vi "Leak check durchfuehren.vi"(8 "TablePictures Refnum In":refnum<vi>[](array[refnum]), 9 "Temperatur":sgl, 10 "Druck FT-IR":sgl, 11 "Aktion":T1) -> (0 "Verstrichene Zeit":sgl, 1 "Druckanstieg":sgl, 2 "Status":string, 3 "Aktion":T1, 4 "Fehler":bool, 5 "Fertig":bool)   [LabVIEW 2020, in "EPA 1065.lvlib" / "Dichtheitstest 1065-345.lvlib"]
uses:
  Dichtheitstest 1065-345.lvlib
  Aktion Leak check durchfuehren.ctl
  Aktion Leak Daten.ctl
  Aktion Protokolldaten_Leak check.ctl
  Sprachverwaltung/FGV Aktion Tabelle zerlegen.ctl
  Funktionstasten/Freigabe Aktionen.ctl
  PNS/Aktionen FGV Grenzwerte.ctl
  Funktionstasten/Zustaende.ctl
  Funktionstasten/Funktionstasten-Aktion.ctl
  Stoerungen/Stoerungen Messgeraet/Aktionen Kommunikation Stoerung.ctl
  Aktion FGV Automatic start.ctl
  Leak Daten.ctl
  Seiten/FT-IR/FT-IR.lvlib
  Stoerungen/Stoerungen.lvlib
  PNS/PNS.lvlib
  Funktionstasten/Funktionstasten.lvlib
  Sprachverwaltung/Sprachverwaltung.lvlib
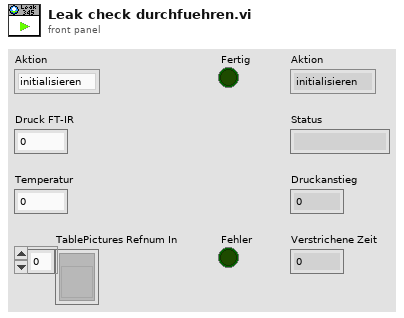
[diagram p1: front panel]
types:
  T1 = typedef "EPA 1065.lvlib/Dichtheitstest 1065-345.lvlib/Aktion Leak check durchfuehren.ctl" = enum16{"initialisieren", "Unterdruck erzeugen", "Ventile schließen", "Warten", "Auswertung", "fertig", "PDF erstellen", "abbrechen"}
  T2 = typedef "EPA 1065.lvlib/Dichtheitstest 1065-345.lvlib/Aktion Leak Daten.ctl" = enum16{"lesen", "laden", "speichern", "Volumen", "berechnen", "Leak check aktiv", "Leak Zustand", "Pfad", "Pfad speichern"}
  T3 = typedef "PNS.lvlib/Aktionen FGV Grenzwerte.ctl" = enum16{"lesen", "Grenzw. schreiben", "Anweisungscode", "IP-Adresse", "laden", "speichern", "Anweisungscode vorgeben"}
  T4 = typedef "Funktionstasten.lvlib/Freigabe Aktionen.ctl" = enum16{"prüfen", "Freigabe?", "lesen"}
  T5 = typedef "Sprachverwaltung.lvlib/FGV Aktion Tabelle zerlegen.ctl" = enum16{"laden", "vereinzeln", "speichern"}
  T6 = typedef "EPA 1065.lvlib/Dichtheitstest 1065-345.lvlib/Aktion Protokolldaten_Leak check.ctl" = enum16{"lesen", "Zeitstempel", "Bearbeiter", "Daten", "Auswertung", "löschen"}
  T7 = typedef "Funktionstasten.lvlib/Funktionstasten-Aktion.ctl" = enum16{"Initialisieren", "Zustand setzen", "Taste gedrückt", "Fehler speichern", "Lesen", "Manuell", "Remote", "Bitparallel", "Samplepoint", "Zeit Prüfen", "reset Umschalten"}
  T8 = typedef "Funktionstasten.lvlib/Zustaende.ctl" = enum16{"Standby", "Pause", "Eco", "Messen", "Kalibrieren", "Spülen Filter", "Spülen Leitung", "Umgebungsluft", "0-Gas", "Cal-Gas", "CG zu PNS", "-------------", "Init 1", "Init 2", "Init 3", "Init 4", "Messen vorbereiten", "Messen durchführen", "Exit"}
  T9 = typedef "EPA 1065.lvlib/Dichtheitstest 1065-345.lvlib/Leak Daten.ctl" = cluster{"Gesamtes Volumen":sgl, "p 1":sgl, "p 2":sgl, "T 1":sgl, "T 2":sgl, "t 1":timestamp, "t 2":timestamp, "Ergebnis mol/s":sgl, "Grenze mol/s":sgl, "Leak in %":sgl, "Ergebnis mbar":sgl, "Grenze mbar":sgl}
  T10 = typedef "EPA 1065.lvlib/Dichtheitstest 1065-345.lvlib/Aktion FGV Automatic start.ctl" = enum16{"lesen", "Test starten aktiv", "Test starten inaktiv", "Seite merken", "Seite zurücksetzen", "AK Start inaktiv"}
  T11 = typedef "Stoerungen.lvlib/Aktionen Kommunikation Stoerung.ctl" = enum16{"lesen", "init", "FT-IR Komm", "FT-IR Betriebsart", "FT-IR Hintergrund", "cRIO Komm", "PNS Komm", "Dichtheitstest", "Life Bit", "FTIR Komm AK", "PMA Komm", "FID Komm", "PMA Cal", "FID Ch4 Cal", "FID THC Cal", "Cal Timeout", "VFS 1 Komm", "VFS 2 Komm", "VFS 3 Komm", "VFS 4 Komm", "TRE 08 Komm", "CG-Test vorzeitig", "CG-Test Span 1", "CG-Test Span 2", "CG-Test Span 3", "CG-Test Messgas", "CG-Test löschen", "Test", "Amium AK", "AK Recept konfig", "AK Name konfig", "AK EKFG konfig"}
  T12 = typedef "EPA 1065.lvlib/Dichtheitstest 1065-345.lvlib/Gesamtvolumen.ctl" = cluster{"FAS":sgl, "d von HL zu VFS":sgl, "l von HL zu VFS":sgl, "VFS":sgl, "d von HL zu SP":sgl, "l von HL zu SP":sgl, "Heizleitung zum VFS":bool, "VFS a":bool, "Heizleitung zur Entnahmestelle":bool, "Gesamtes Volumen":sgl, "LeakValve":u16, "Einheit":enum16{"mol/s", "mbar"}}
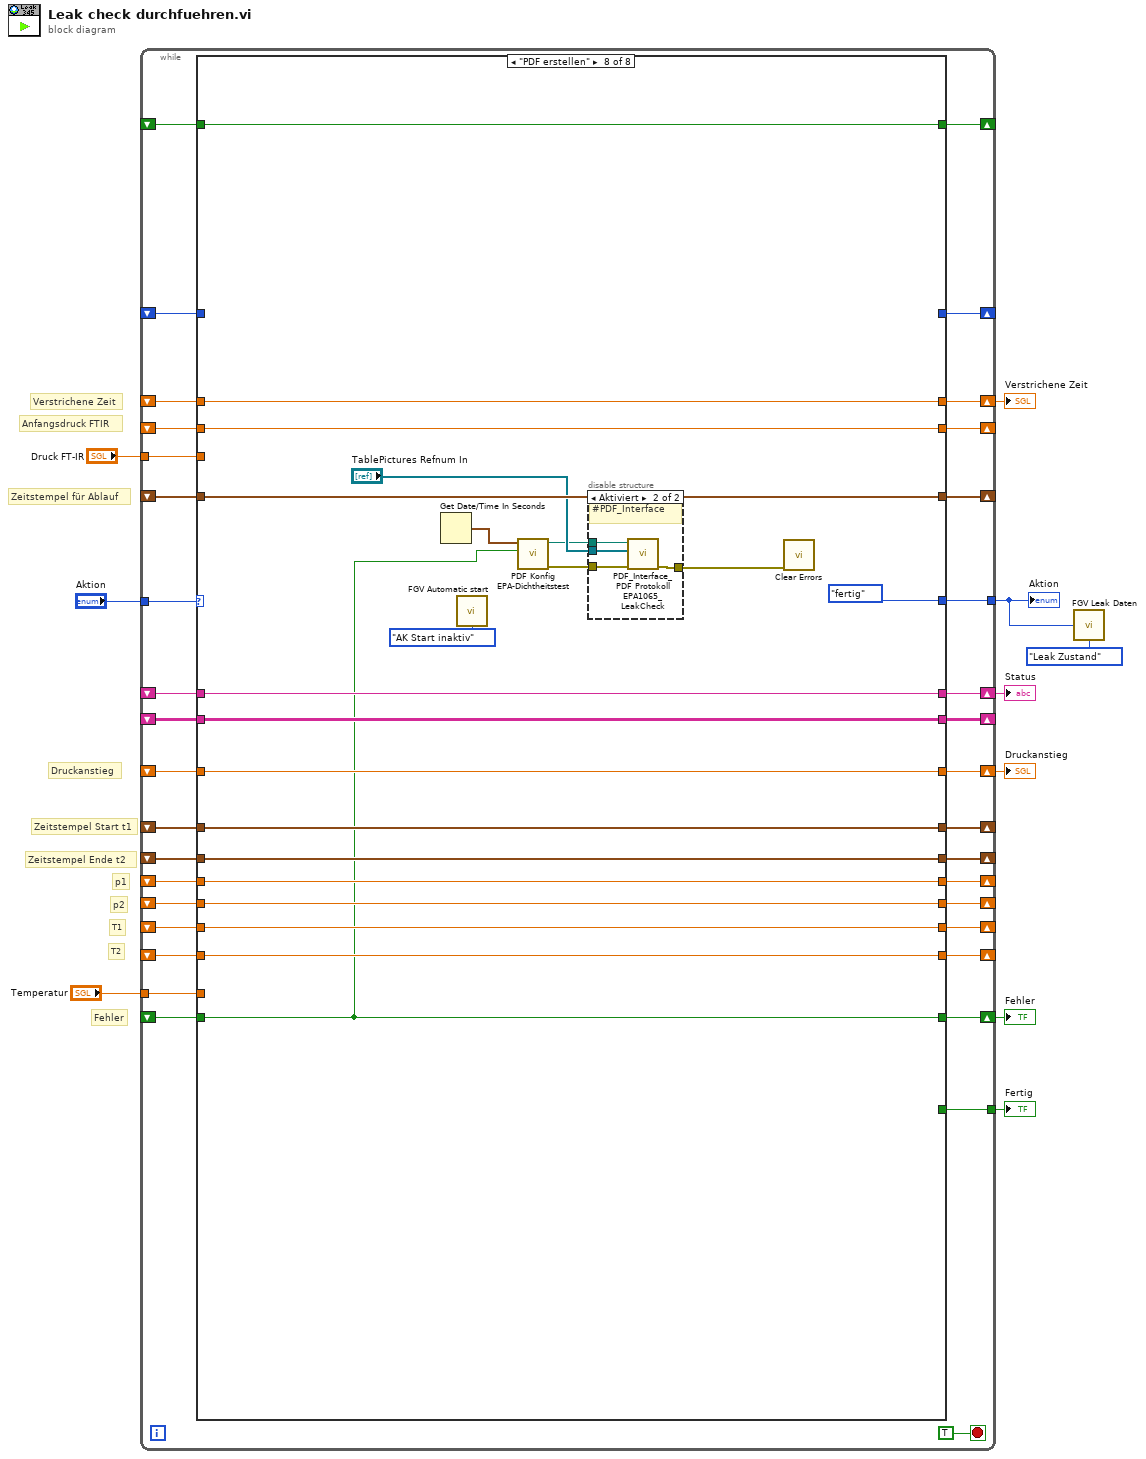
[diagram p0: block diagram]
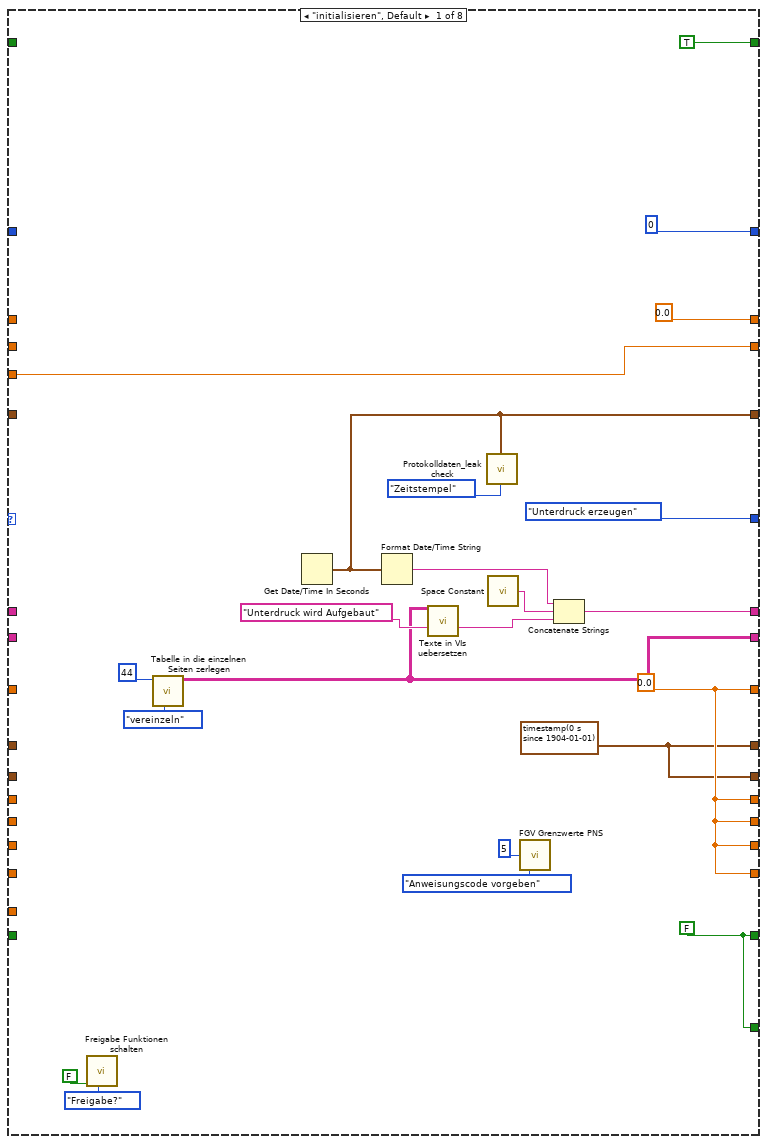
[diagram p2: hidden frame]
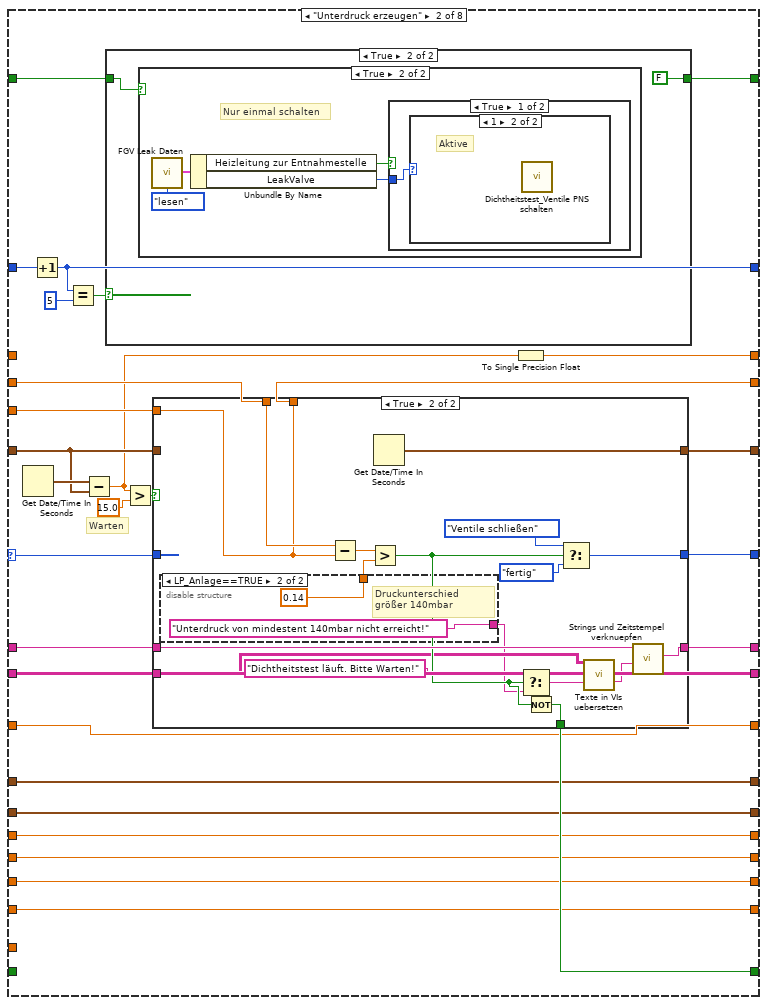
[diagram p3: hidden frame]
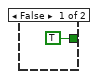
[diagram p4: hidden frame]
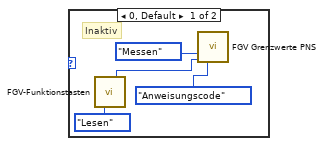
[diagram p6: hidden frame]
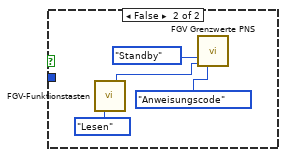
[diagram p7: hidden frame]
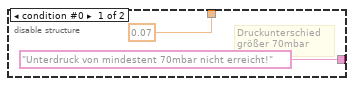
[diagram p9: hidden frame]
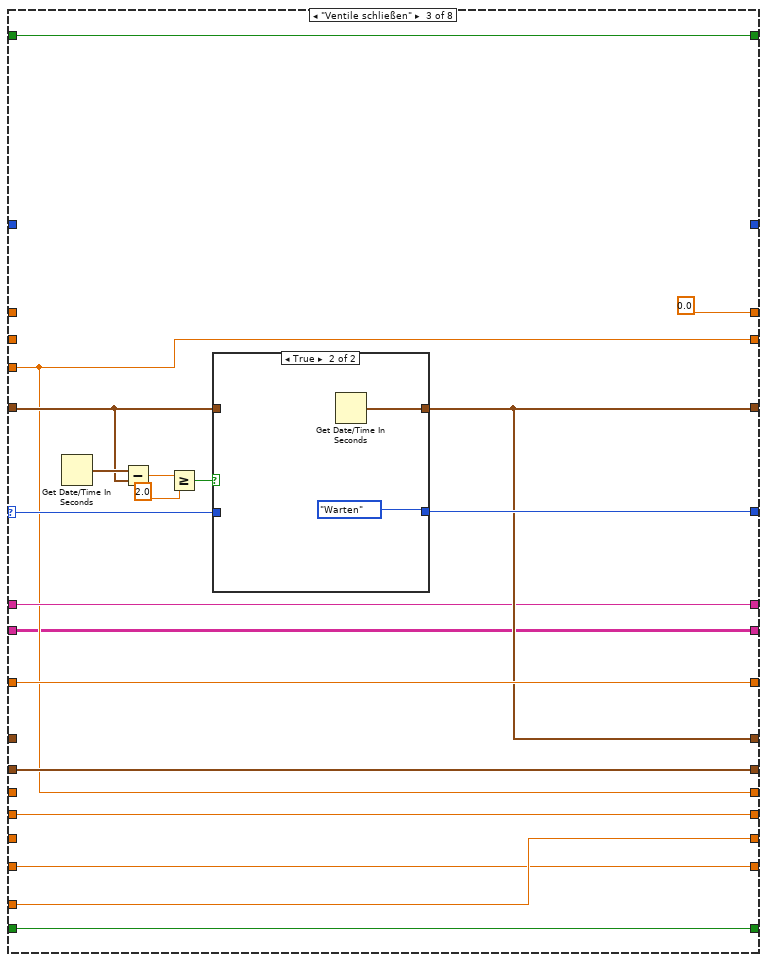
[diagram p10: hidden frame]
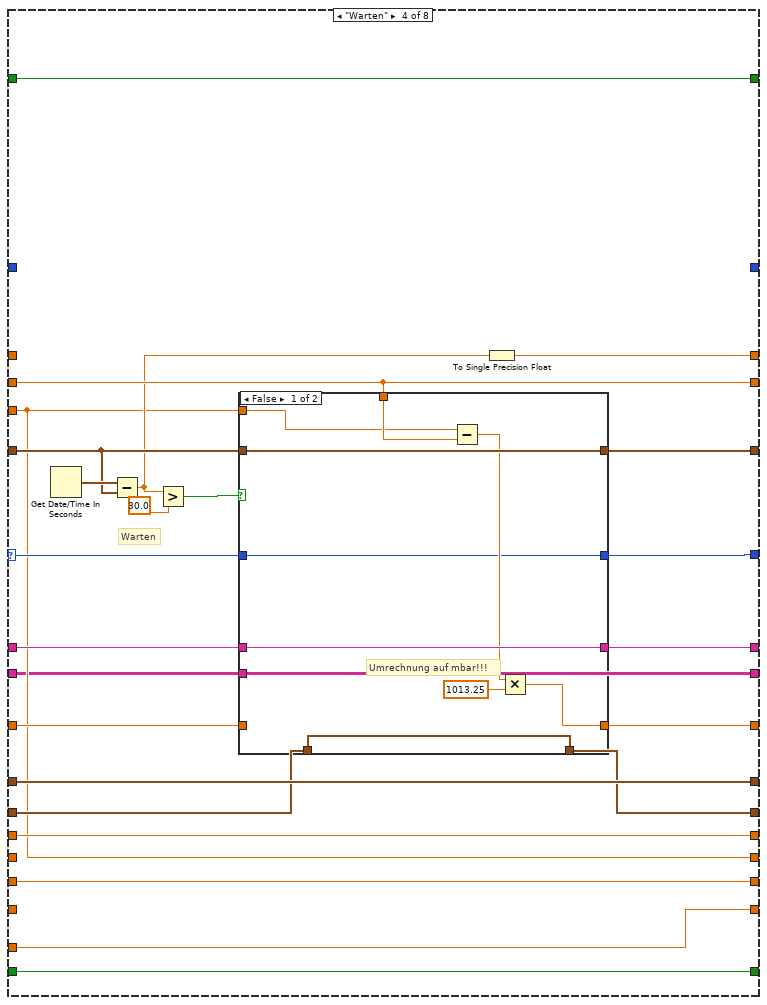
[diagram p12: hidden frame]
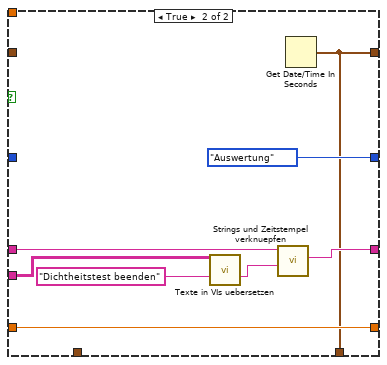
[diagram p13: hidden frame]
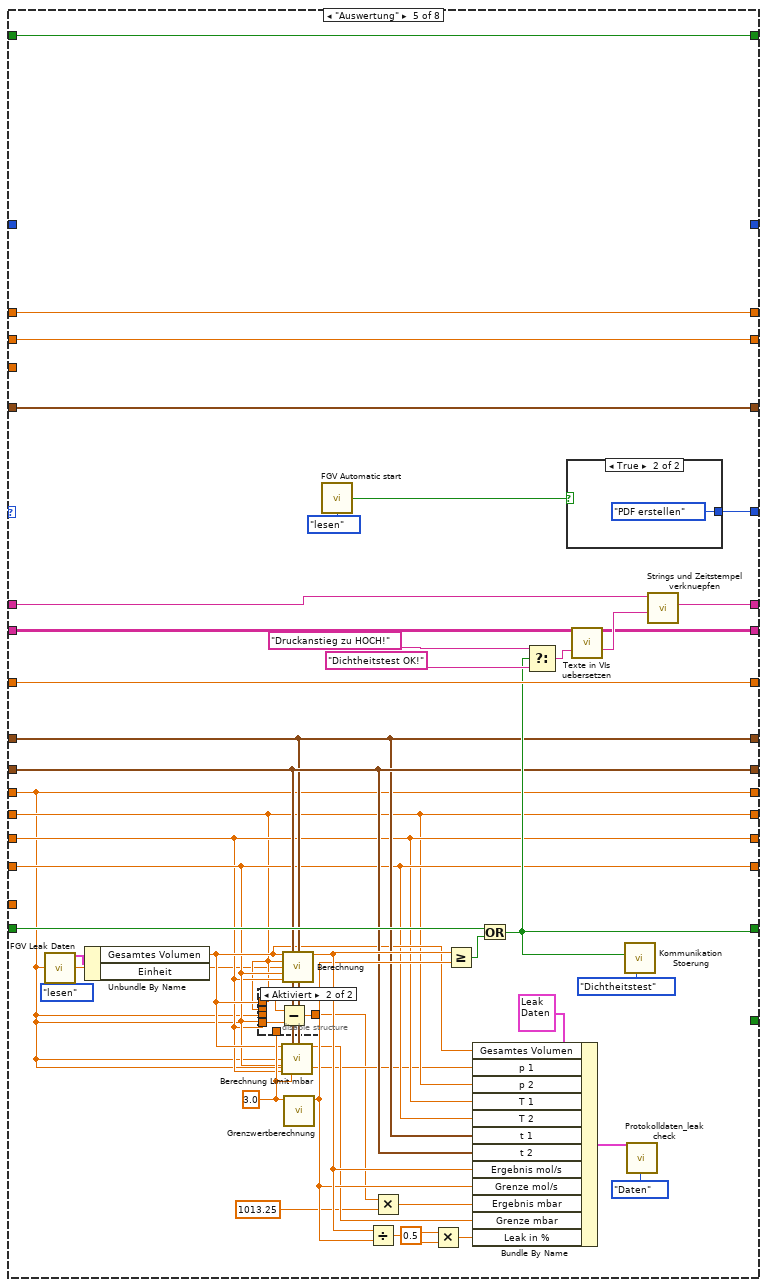
[diagram p14: hidden frame]
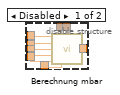
[diagram p15: hidden frame]
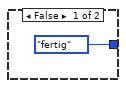
[diagram p16: hidden frame]
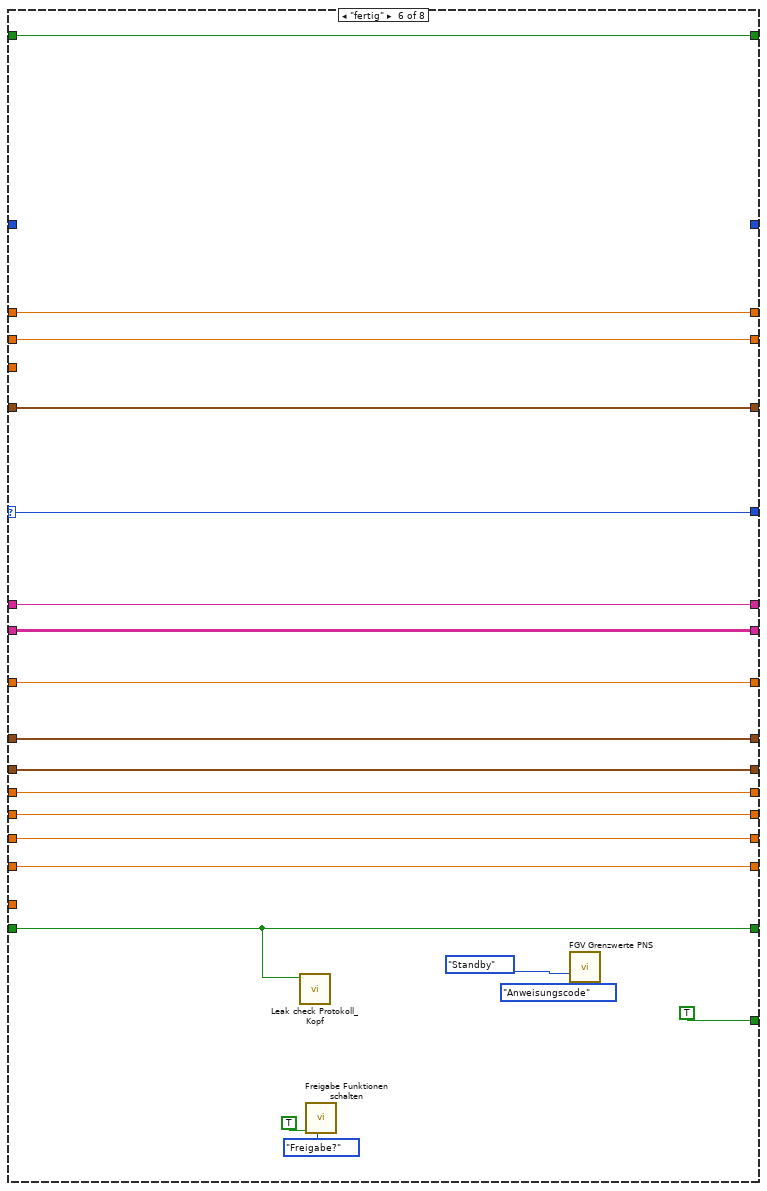
[diagram p17: hidden frame]
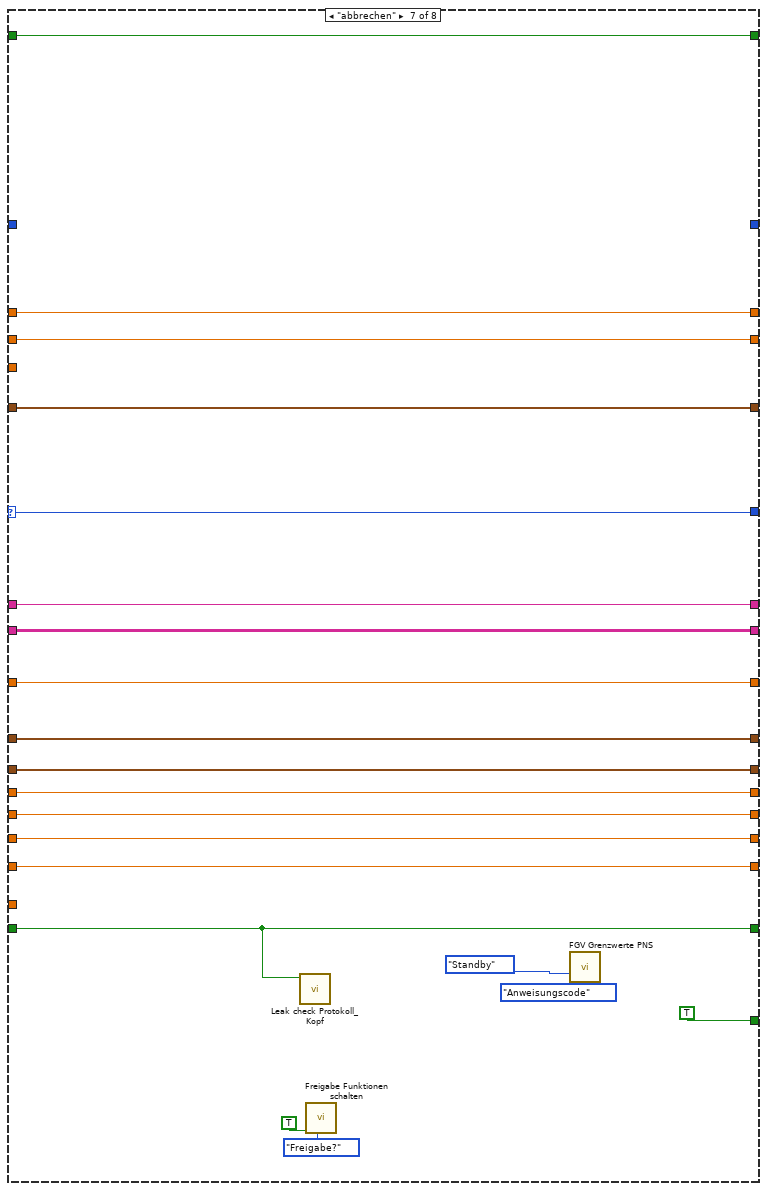
[diagram p18: hidden frame]
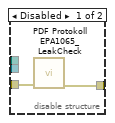
[diagram p19: hidden frame]
diagram:
  # "T2"
  # "T1"
  # "p2"
  # "p1"
  # "Druckanstieg"
  # "Zeitstempel Ende t2"
  # "Zeitstempel Start t1"
  # "Fehler"
  # "Zeitstempel für Ablauf"
  # "Verstrichene Zeit"
  # "Anfangsdruck FTIR"
  n1 = while {
    shift-right: [w44] -> _
    shift-left: _ -> [w42]
    shift-right: [w41] -> w8
    shift-left: _ -> [w40]
    tunnel: "Aktion" -> [w45]
    tunnel: [w43] -> w1
    tunnel: "Druck FT-IR" -> [w39]
    shift-right: [w38] -> _
    shift-left: _ -> [w37]
    shift-right: [w36] -> w6
    shift-left: _ -> [w35]
    shift-right: [w34] -> w4
    shift-left: _ -> [w33]
    shift-right: [w32] -> w5
    shift-left: _ -> [w31]
    shift-right: [w30] -> _
    shift-left: _ -> [w29]
    shift-right: [w27] -> _
    shift-left: _ -> [w28]
    shift-right: [w26] -> _
    shift-left: _ -> [w25]
    shift-right: [w24] -> _
    shift-left: _ -> [w23]
    tunnel: "Temperatur" -> [w22]
    shift-right: [w21] -> _
    shift-left: _ -> [w20]
    shift-right: [w19] -> _
    shift-left: _ -> [w18]
    tunnel: [w17] -> w3
    shift-right: [w16] -> _
    shift-left: _ -> [w15]
    shift-right: [w14] -> _
    shift-left: _ -> [w13]
    shift-right: [w12] -> _
    shift-left: _ -> [w11]
    stop <- TRUE stop-if-true
    n2 = case shown="\"PDF erstellen\"" w45 {
      selector: w45 -> [_ w90 w152 w178 _ w274 w294 _]
      tunnel: [w58 w97 w150 w184 w241 w275 w295 w316] -> w44
      tunnel: [Aktion_Leak_check_durchfuehren."Unterdruck erzeugen" ("Aktion") w89 w151 w177 w238 w274 w294 Aktion_Leak_check_durchfuehren."fertig" ("Aktion")] -> w43
      tunnel: w42 -> [_ w93 w153 w182 w241 w275 w295 w316]
      tunnel: [w65 w92 w147 w175 w232 w273 w293 w314] -> w41
      tunnel: w40 -> [_ w91 w147 w176 w233 w273 w293 w314]
      tunnel: w39 -> [w64 w88 w145 w167 _ _ _ _]
      tunnel: [w64 w86 w145 w180 w240 w276 w296 w317] -> w38
      tunnel: w37 -> [_ w87 _ w180 w240 w276 w296 w317]
      tunnel: [sgl 0.0 w77 sgl 0.0 w164 w239 w277 w297 w318] -> w36
      tunnel: w35 -> [_ _ _ _ w239 w277 w297 w318]
      tunnel: [w60 w85 w141 w169 w229 w262 w282 w302] -> w34
      tunnel: w33 -> [_ _ w141 w169 w234 w262 w282 w302]
      tunnel: [w62 w82 w157 w174 w242 w272 w292 w312] -> w32
      tunnel: w31 -> [_ w82 w157 w173 w242 w272 w292 w312]
      tunnel: [w61 w84 w150 w172 w212 w271 w291 w311] -> w30
      tunnel: w29 -> [_ w84 _ w172 w212 w271 w291 w311]
      tunnel: w28 -> [_ w83 w149 w170 w213 w270 w290 w310]
      tunnel: [w61 w83 w149 w171 w213 w270 w290 w310] -> w27
      tunnel: [w62 w81 w145 w168 w206 w269 w289 w309] -> w26
      tunnel: w25 -> [_ w81 _ w168 w206 w269 w289 w309]
      tunnel: [w62 w80 w143 w167 w207 w268 w288 w308] -> w24
      tunnel: w23 -> [_ w80 w143 _ w207 w268 w288 w308]
      tunnel: w22 -> [_ _ w144 w166 _ _ _ _]
      tunnel: [w62 w78 w142 w166 w210 w266 w286 w306] -> w21
      tunnel: w20 -> [_ w78 w142 _ w210 w266 w286 w306]
      tunnel: [w62 w79 w144 w165 w209 w267 w287 w307] -> w19
      tunnel: w18 -> [_ w79 _ w165 w209 w267 w287 w307]
      tunnel: [w60 _ _ _ _ TRUE TRUE _] -> w17
      tunnel: [w54 w76 w140 w163 w225 w261 w281 w313] -> w16
      tunnel: w15 -> [_ w76 w140 w163 w225 w261 w281 w313]
      tunnel: [0 w73 _ _ _ _ _ _] -> w14
      tunnel: w13 -> [_ w74 _ _ _ _ _ _]
      tunnel: [TRUE w70 w139 w162 w220 w258 w278 w300] -> w12
      tunnel: w11 -> [_ w69 w139 w162 w220 w258 w278 w300]
      frame "initialisieren", Default {
        w60 = FALSE
        w61 = timestamp(0 s since 1904-01-01) ("seconds since 1Jan1904")
        w62 = sgl 0.0
        n3 = call "Freigabe Funktionen schalten.vi"("Aktionen"=Freigabe_Aktionen."Freigabe?", "Freigabe?"=FALSE) -> ()  [unwired: 7 in, 3 out]
        n4 = call "Tabelle in die einzelnen Seiten zerlegen.vi"("Aktion"=FGV_Aktion_Tabelle_zerlegen."vereinzeln", "Index (Seite)"=44) -> ("Sprachliste"=w54:string[][])  [unwired: 7 in, 2 out]
        n5 = Get Date/Time In Seconds() -> (seconds since 1Jan1904=w58:timestamp)
        n6 = Format Date/Time String(seconds (now)=w58) -> (date/time string=w68:string)  [unwired: 2 in]
        n7 = call "Texte in VIs uebersetzen.vi"("Sprachliste"=w54, "String zum Übersetzen"="Unterdruck wird Aufgebaut" ("String")) -> ("String zum Übersetzen"=w55:string)  [unwired: 9 in, 4 out]
        n8 = call "Protokolldaten_leak check.vi"("Start"=w58, "Aktion"=Aktion_Protokolldaten_Leak_check."Zeitstempel") -> ()  [unwired: 22 in, 4 out]
        n9 = call <vilib>:"Space Constant.vi"() -> ("String"=w67:string)
        n10 = call "FGV Grenzwerte PNS.vi"("Anweisungscode"=u16 5, "Aktionen FGV Grenzwerte"=Aktionen_FGV_Grenzwerte."Anweisungscode vorgeben") -> ()  [unwired: 11 in, 3 out]
        n11 = Concatenate Strings(w68, w67, w55) -> (w65:string)
      }
      frame "Unterdruck erzeugen" {
        # "Warten"
        n12 = Get Date/Time In Seconds() -> (seconds since 1Jan1904=w95:timestamp)
        n13 = Increment(x=w74) -> (x+1=w73:i32)
        n14 = Equal?(x=w73, y=5) -> (x = y?=w71:bool)
        n15 = Subtract(x=w95, y=w93) -> (x-y=w75:dbl)
        n16 = case shown="True" w71 {
          tunnel: [TRUE FALSE] -> w70
          tunnel: w69 -> [_ w99]
          frame False {
          }
          frame True {
            n17 = case shown="True" w99 {
              frame False {
              }
              frame True {
                # "Nur einmal schalten"
                n18 = call "FGV Leak Daten.vi"("Aktion"=Aktion_Leak_Daten."lesen") -> ("Gesamtvolumen"=w103:T12)  [unwired: 10 in, 4 out]
                n19 = Unbundle By Name(w103) -> ("Heizleitung zur Entnahmestelle"=w102:bool, "LeakValve"=w101:u16)
                n20 = case shown="True" w102 {
                  tunnel: w101 -> [w105 _]
                  frame True {
                    n21 = case shown="1" w105 {
                      frame 0, Default {
                        # "Inaktiv"
                        n22 = call "FGV-Funktionstasten.vi"("Aktion"=Funktionstasten-Aktion."Lesen") -> ("Samplepoint"=w106:u16)  [unwired: 7 in, 7 out]
                        n23 = call "FGV Grenzwerte PNS.vi"("Zustand"=Zustaende."Messen", "Samplepoint"=w106, "Aktionen FGV Grenzwerte"=Aktionen_FGV_Grenzwerte."Anweisungscode") -> ()  [unwired: 10 in, 3 out]
                      }
                      frame 1 {
                        # "Aktive"
                        n24 = call "Dichtheitstest_Ventile PNS schalten.vi"() -> ()  [unwired: 11 in, 1 out]
                      }
                    }
                  }
                  frame False {
                    n25 = call "FGV-Funktionstasten.vi"("Aktion"=Funktionstasten-Aktion."Lesen") -> ("Samplepoint"=w110:u16)  [unwired: 7 in, 7 out]
                    n26 = call "FGV Grenzwerte PNS.vi"("Zustand"=Zustaende."Standby", "Samplepoint"=w110, "Aktionen FGV Grenzwerte"=Aktionen_FGV_Grenzwerte."Anweisungscode") -> ()  [unwired: 10 in, 3 out]
                  }
                }
              }
            }
          }
        }
        n27 = Greater?(x=w75, y=15.0) -> (0:w94:bool)
        n28 = case shown="True" w94 {
          tunnel: w93 -> [w117 _]
          tunnel: [w117 w122] -> w97
          tunnel: w87 -> [w116 w134]
          tunnel: [w116 w125] -> w86
          tunnel: [w115 w131] -> w89
          tunnel: w91 -> [w114 w130]
          tunnel: [w114 w129] -> w92
          tunnel: w90 -> [w115 _]
          tunnel: [_ w126] -> w85
          tunnel: w88 -> [_ w125]
          tunnel: w76 -> [_ w119]
          frame False {
          }
          frame True {
            n29 = disable-structure shown="LP_Anlage==TRUE" {
              disable-tunnel: [0.07 ("y") 0.14 ("y")] -> w132
              disable-tunnel: ["Unterdruck von mindestent 70mbar nicht erreicht!" ("String") "Unterdruck von mindestent 140mbar nicht erreicht!" ("String")] -> w118
              frame condition #0 {
                # "Druckunterschied \ngrößer 70mbar"
              }
              frame condition #1 (active) {
                # "Druckunterschied \ngrößer 140mbar"
              }
            }
            n30 = Subtract(x=w134, y=w125) -> (x-y=w133:sgl)
            n31 = Greater?(x=w133, y=w132) -> (0:w127:bool)
            n32 = Get Date/Time In Seconds() -> (seconds since 1Jan1904=w122:timestamp)
            n33 = Select(t="Dichtheitstest läuft. Bitte Warten!" ("String"), s=w127, f=w118) -> (s? t:f=w120:string)
            n34 = Not(x=w127) -> (.not. x?=w126:bool)
            n35 = Select(t=Aktion_Leak_check_durchfuehren."Ventile schließen", s=w127, f=Aktion_Leak_check_durchfuehren."fertig" ("Aktion")) -> (s? t:f=w131:T1)
            n36 = call "Texte in VIs uebersetzen.vi"("Sprachliste"=w119, "String zum Übersetzen"=w120) -> ("String zum Übersetzen"=w121:string)  [unwired: 9 in, 4 out]
            n37 = call "Strings und Zeitstempel verknuepfen.vi"("String 1 hinzufügen"=w121, "Eingagns String"=w130) -> ("Verknüpfter String"=w129:string)  [unwired: 9 in]
          }
        }
        n38 = To Single Precision Float(number=w75) -> (single precision float=w77:sgl)
      }
      frame "Ventile schließen" {
        n39 = Get Date/Time In Seconds() -> (seconds since 1Jan1904=w154:timestamp)
        n40 = Subtract(x=w154, y=w153) -> (x-y=w155:dbl)
        n41 = Greater Or Equal?(x=w155, y=2.0) -> (x >= y?=w146:bool)
        n42 = case shown="True" w146 {
          tunnel: w153 -> [w159 _]
          tunnel: w152 -> [w158 _]
          tunnel: [w158 Aktion_Leak_check_durchfuehren."Warten" ("t")] -> w151
          tunnel: [w159 w160] -> w150
          frame False {
          }
          frame True {
            n43 = Get Date/Time In Seconds() -> (seconds since 1Jan1904=w160:timestamp)
          }
        }
      }
      frame "Warten" {
        # "Warten"
        n44 = Get Date/Time In Seconds() -> (seconds since 1Jan1904=w185:timestamp)
        n45 = Subtract(x=w185, y=w182) -> (x-y=w179:dbl)
        n46 = Greater?(x=w179, y=30.0) -> (0:w183:bool)
        n47 = case shown="False" w183 {
          tunnel: w182 -> [w194 _]
          tunnel: [w194 w198] -> w184
          tunnel: w178 -> [w187 _]
          tunnel: w176 -> [w193 w202]
          tunnel: w173 -> [_ w201]
          tunnel: [w191 w201] -> w174
          tunnel: [w193 w200] -> w175
          tunnel: w180 -> [w189 _]
          tunnel: w167 -> [w188 _]
          tunnel: [w187 Aktion_Leak_check_durchfuehren."Auswertung" ("Aktion")] -> w177
          tunnel: [w186 w198] -> w171
          tunnel: w170 -> [w186 _]
          tunnel: w163 -> [_ w195]
          frame False {
            # "Umrechnung auf mbar!!!"
            n48 = Subtract(x=w188, y=w189) -> (x-y=w190:sgl)
            n49 = Multiply(x=w190, y=sgl 1013.25) -> (x*y=w191:sgl)
          }
          frame True {
            n50 = call "Texte in VIs uebersetzen.vi"("Sprachliste"=w195, "String zum Übersetzen"="Dichtheitstest beenden" ("String")) -> ("String zum Übersetzen"=w196:string)  [unwired: 9 in, 4 out]
            n51 = call "Strings und Zeitstempel verknuepfen.vi"("String 1 hinzufügen"=w196, "Eingagns String"=w202) -> ("Verknüpfter String"=w200:string)  [unwired: 9 in]
            n52 = Get Date/Time In Seconds() -> (seconds since 1Jan1904=w198:timestamp)
          }
        }
        n53 = To Single Precision Float(number=w179) -> (single precision float=w164:sgl)
      }
      frame "Auswertung" {
        w214 = sgl 3.0 ("Durchfluss")
        n54 = call "FGV Leak Daten.vi"("Aktion"=Aktion_Leak_Daten."lesen") -> ("Gesamtvolumen"=w236:T12)  [unwired: 10 in, 4 out]
        n55 = Unbundle By Name(w236) -> ("Gesamtes Volumen"=w211:sgl)  [unwired: 1 out]
        n56 = disable-structure shown="Aktiviert" {
          disable-tunnel: w207 -> [w252 _]
          disable-tunnel: [w251 w255] -> w205
          disable-tunnel: w214 -> [w250 _]
          disable-tunnel: w213 -> [w249 _]
          disable-tunnel: w212 -> [w248 _]
          disable-tunnel: w211 -> [w247 _]
          disable-tunnel: w206 -> [w246 _]
          disable-tunnel: w210 -> [w245 _]
          disable-tunnel: w209 -> [w244 _]
          disable-tunnel: w207 -> [_ w254]
          disable-tunnel: w206 -> [_ w253]
          frame Disabled {
            n57 = call "Berechnung mbar.vi"("Volumen in mm³"=w247, "t2"=w249, "t1"=w248, "p2"=w252, "p1"=w246, "T2 in C°"=w245, "T1 in C°"=w244, "Fluss in l/min"=w250) -> ("n in mbar"=w251:sgl)  [unwired: 7 in]
          }
          frame Enabled {
            n58 = Subtract(x=w254, y=w253) -> (x-y=w255:sgl)
          }
        }
        n59 = call "Berechnung Limit mbar.vi"("Volumen in mm³"=w211, "t2"=w213, "t1"=w212, "p1"=w206, "T2 in C°"=w210, "T1 in C°"=w209, "Fluss in l/min"=w214) -> ("Limit in mbar"=w208:sgl)  [unwired: 7 in, 1 out]
        n60 = call "Berechnung.vi"("Volumen in mm³"=w211, "t2"=w213, "t1"=w212, "p2"=w207, "p1"=w206, "T2 in C°"=w210, "T1 in C°"=w209) -> ("n"=w218:sgl)  [unwired: 8 in]
        n61 = call "Grenzwertberechnung.vi"("Durchfluss"=w214) -> ("Grenze"=w217:sgl)  [unwired: 10 in]
        n62 = call "FGV Automatic start.vi"("Aktion"=Aktion_FGV_Automatic_start."lesen") -> ("AK Start"=w223:bool)  [unwired: 12 in, 2 out]
        n63 = Divide(x=w218, y=w217) -> (x/y=w222:sgl)
        n64 = Multiply(x=w205, y=sgl 1013.25) -> (x*y=w204:sgl)
        n65 = Multiply(x=w222, y=sgl 0.5) -> (x*y=w215:sgl)
        n66 = Greater Or Equal?(x=w218, y=w217) -> (x >= y?=w235:bool)
        n67 = Bundle By Name(cluster=T9 {"Gesamtes Volumen"=0.0, "p 1"=0.0, "p 2"=0.0, "T 1"=0.0, "T 2"=0.0, "t 1"=timestamp(0 s since 1904-01-01), "t 2"=timestamp(0 s since 1904-01-01), "Ergebnis mol/s"=0.0, "Grenze mol/s"=0.0, "Leak in %"=0.0, "Ergebnis mbar"=0.0, "Grenze mbar"=0.0} ("Daten"), "Gesamtes Volumen"=w211, "p 1"=w206, "p 2"=w207, "T 1"=w209, "T 2"=w210, "t 1"=w212, "t 2"=w213, "Ergebnis mol/s"=w218, "Grenze mol/s"=w217, "Ergebnis mbar"=w204, "Grenze mbar"=w208, "Leak in %"=w215) -> (w216:T9)
        n68 = Or(x=w234, y=w235) -> (x .or. y?=w229:bool)
        n69 = Select(t="Druckanstieg zu HOCH!" ("String"), s=w229, f="Dichtheitstest OK!" ("String")) -> (s? t:f=w227:string)
        n70 = case shown="True" w223 {
          tunnel: [Aktion_Leak_check_durchfuehren."fertig" ("Aktion") Aktion_Leak_check_durchfuehren."PDF erstellen" ("Aktion")] -> w238
          frame False {
          }
          frame True {
          }
        }
        n71 = call "Texte in VIs uebersetzen.vi"("Sprachliste"=w225, "String zum Übersetzen"=w227) -> ("String zum Übersetzen"=w226:string)  [unwired: 9 in, 4 out]
        n72 = call "Kommunikation Stoerung.vi"("Aktionen"=Aktionen_Kommunikation_Stoerung."Dichtheitstest", "ERROR"=w229) -> ()  [unwired: 9 in, 1 out]
        n73 = call "Protokolldaten_leak check.vi"("Daten"=w216, "Aktion"=Aktion_Protokolldaten_Leak_check."Daten") -> ()  [unwired: 22 in, 4 out]
        n74 = call "Strings und Zeitstempel verknuepfen.vi"("String 1 hinzufügen"=w226, "Eingagns String"=w233) -> ("Verknüpfter String"=w232:string)  [unwired: 9 in]
      }
      frame "fertig" {
        n75 = call "Leak check Protokoll_Kopf.vi"("Externer Fehler"=w262) -> ()  [unwired: 11 in]
        n76 = call "Freigabe Funktionen schalten.vi"("Aktionen"=Freigabe_Aktionen."Freigabe?", "Freigabe?"=TRUE) -> ()  [unwired: 7 in, 3 out]
        n77 = call "FGV Grenzwerte PNS.vi"("Zustand"=Zustaende."Standby", "Aktionen FGV Grenzwerte"=Aktionen_FGV_Grenzwerte."Anweisungscode") -> ()  [unwired: 11 in, 3 out]
      }
      frame "abbrechen" {
        n78 = call "Leak check Protokoll_Kopf.vi"("Externer Fehler"=w282) -> ()  [unwired: 11 in]
        n79 = call "Freigabe Funktionen schalten.vi"("Aktionen"=Freigabe_Aktionen."Freigabe?", "Freigabe?"=TRUE) -> ()  [unwired: 7 in, 3 out]
        n80 = call "FGV Grenzwerte PNS.vi"("Zustand"=Zustaende."Standby", "Aktionen FGV Grenzwerte"=Aktionen_FGV_Grenzwerte."Anweisungscode") -> ()  [unwired: 11 in, 3 out]
      }
      frame "PDF erstellen" {
        n81 = Get Date/Time In Seconds() -> (seconds since 1Jan1904=w303:timestamp)
        n82 = call "FGV Automatic start.vi"("Aktion"=Aktion_FGV_Automatic_start."AK Start inaktiv") -> ()  [unwired: 12 in, 3 out]
        n83 = call "PDF Konfig EPA-Dichtheitstest.vi"("Failed"=w302, "seconds since 1Jan1904"=w303) -> ("error out"=w301:errorcluster, "PDF Pfad"=w298:path)  [unwired: 8 in]
        n84 = disable-structure shown="Aktiviert" {
          disable-tunnel: [w320 w323] -> w304
          disable-tunnel: w301 -> [w319 w324]
          disable-tunnel: "TablePictures Refnum In" -> [_ w322]
          disable-tunnel: w298 -> [_ w321]
          frame Disabled {
            n85 = call "PDF Protokoll EPA1065_LeakCheck.vi"("error in (no error)"=w319) -> ("error out"=w320:errorcluster)  [unwired: 10 in]
          }
          frame Enabled {
            # "#PDF_Interface"
            n86 = call "PDF_Interface_PDF Protokoll EPA1065_LeakCheck.vi"("error in (no error)"=w324, "TablePictures Refnum In"=w322, "Save PDF File Path"=w321) -> ("error out"=w323:errorcluster)  [unwired: 8 in]
          }
        }
        n87 = call <vilib>:"Clear Errors.vi"("error in (no error)"=w304) -> ()  [unwired: 5 in, 2 out]
      }
    }
  }
  "Aktion" <- w1
  "Status" <- w8
  "Verstrichene Zeit" <- w6
  "Druckanstieg" <- w5
  "Fehler" <- w4
  "Fertig" <- w3
  n88 = call "FGV Leak Daten.vi"("Dichtheitstest Zustand"=w1, "Aktion"=Aktion_Leak_Daten."Leak Zustand") -> ()  [unwired: 9 in, 5 out]
